vi "Init DAQ Digital Output.vi"(8 "error in":errorcluster, 10 "name to assign":string, 11 "lines":tag="Dev1/port0/line0") -> (0 "error out":errorcluster, 3 "Refnum out":refnum<k21>)   [LabVIEW 2021]
uses:
  <vilib>/DAQmx/create/channels.llb/DAQmx Create Channel (DO-Digital Output).vi
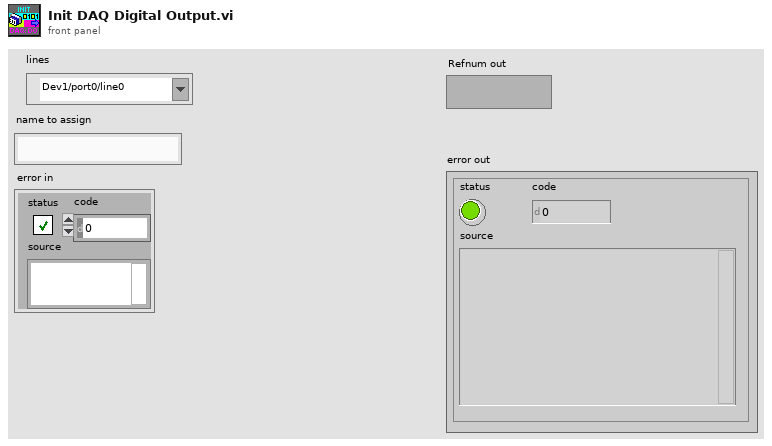
[diagram p1: front panel]
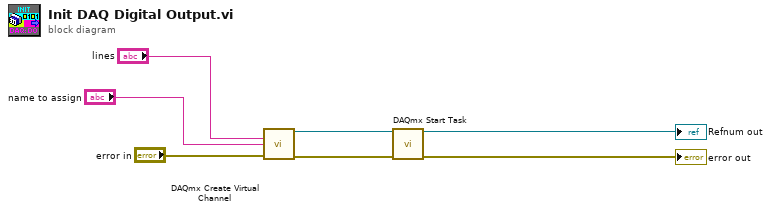
[diagram p0: block diagram]
diagram:
  n1 = call-poly <vilib>:"DAQmx Create Virtual Channel.vi"("lines"="lines", "name to assign"="name to assign", "error in"="error in") -> ("task out"=w5:refnum<k21>, "error out"=w4:errorcluster)  [unwired: 11 in]
  n2 = call <vilib>:"DAQmx Start Task.vi"("task/channels in"=w5, "error in"=w4) -> ("task out"=→"Refnum out":refnum<k21>, "error out"=→"error out":errorcluster)  [unwired: 12 in]
